vi "Get Data Segment.vi"(6 "Offset (-1 default)":i32=-1, 8 "error in (no error)":errorcluster, 9 "Length":i32, 10 "Bytes in":u8[](array[numeric]), 11 "pcap Parse and Build in":refnum<class "pcap_Parse_Build_CIF.lvclass">) -> (0 "error out":errorcluster, 1 "Data Segment":u8[](array[numeric]), 2 "Bytes out":u8[](array[numeric]), 3 "pcap Parse and Build out":refnum<class "pcap_Parse_Build_CIF.lvclass">)   [LabVIEW 2021, in "pcap_Parse_Build_CIF.lvclass"]
doc: "Update the timestamp in-line with the byte array. This is useful for changing time offset of existing data. \n\nIf called after the Parse Packet Header then the offset can be left at the default -1. It will automatically back-up one header set from the current offset. If a value other than -1 is provided it will update the bytes at that location. There is no check to verify location in the byte stream so it is possible to corrupt data if incorrect offsets are used."
uses:
  pcap_Parse_Build_CIF.lvclass
  pcap_Parse_Build_CIF.lvclass/pcap_Parse_Build_CIF.ctl
  Typedef/Errors.ctl
  <vilib>/CIF Foundation/CIF Utilities/Errors/Append Error Location.vi
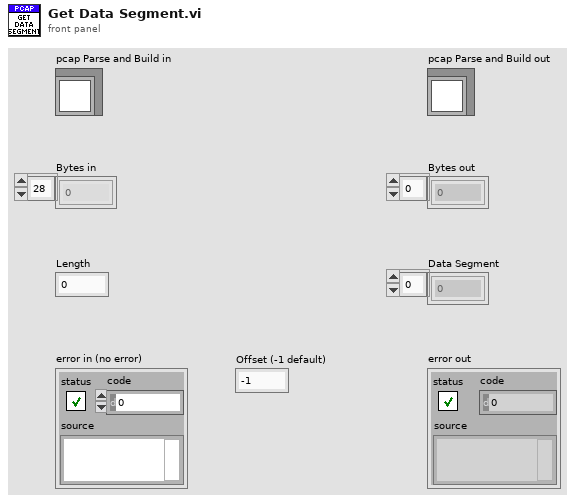
[diagram p1: front panel]
types:
  T1 = typedef "pcap_Parse_Build_CIF.lvclass/Errors.ctl" = enum16{"Invalid Global Header", "Out of Data"}
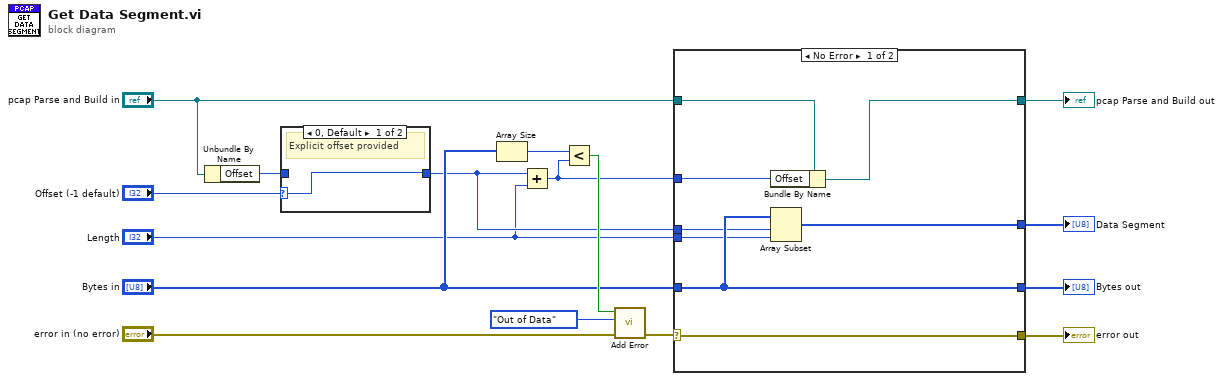
[diagram p0: block diagram]
diagram:
  n1 = Unbundle By Name("pcap Parse and Build in") -> ("Offset"=w1:i32)
  n2 = case shown="0, Default" "Offset (-1 default)" {
    selector: "Offset (-1 default)" -> [w16 _]
    tunnel: w1 -> [_ w17]
    tunnel: [w16 w17] -> w6
    frame 0, Default {
      # "Explicit offset provided"
    }
    frame -1 {
      # "Use existing offset"
    }
  }
  n3 = Array Size(array="Bytes in") -> (size(s)=w9:i32)
  n4 = Add(x=w6, y="Length") -> (x+y=w3:i32)
  n5 = Less?(x=w9, y=w3) -> (x < y?=w11:bool)
  n6 = call "Add Error.vi"("Error"=Errors."Out of Data", "Insert Error"=w11) -> ()  [unwired: 9 in, 1 out]
  n7 = case shown="No Error" "error in (no error)" {
    selector: "error in (no error)" -> [w25 w28]
    tunnel: [w25 w28] -> w14
    tunnel: [w19 w27] -> w12
    tunnel: "pcap Parse and Build in" -> [w21 w27]
    tunnel: "Bytes in" -> [w24 w26]
    tunnel: w6 -> [w23 _]
    tunnel: "Length" -> [w22 _]
    tunnel: [w24 w26] -> w5
    tunnel: w3 -> [w20 _]
    tunnel: [w18 _] -> w2
    frame No Error {
      n8 = Bundle By Name(cluster=w21, "Offset"=w20) -> (w19:refnum<class "pcap_Parse_Build_CIF.lvclass">)
      n9 = Array Subset(array=w24, index=w23, length=w22) -> (w18:u8[])
    }
    frame Error {
    }
  }
  "error out" <- w14
  "pcap Parse and Build out" <- w12
  "Bytes out" <- w5
  "Data Segment" <- w2
